vi "Entry.vi"(8 "error in (no error)":errorcluster, 11 "New State":refnum<class "Command State Actor.lvclass">) -> (0 "error out":errorcluster, 3 "State out":refnum<class "Command State Actor.lvclass">)   [LabVIEW 2013, in "Command State Actor.lvlib" / "Command State Actor.lvclass"]
doc: "This is an abstract method. Override this method to define the behavior when you enter the state."
uses:
  Command State Actor.lvclass
  <vilib>/ni/Actors/State Actor/State Actor/State Actor.lvclass
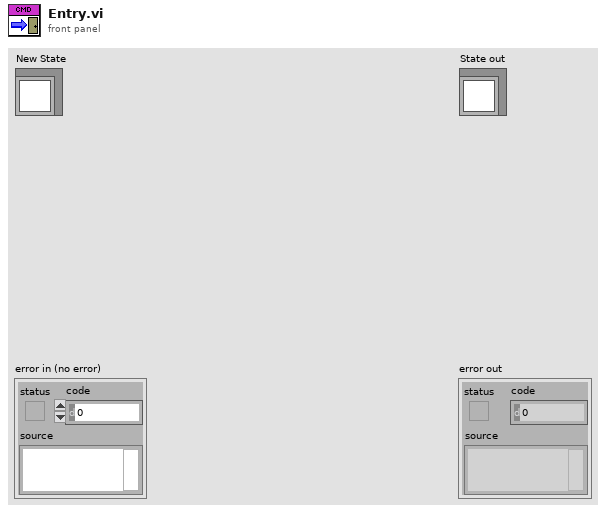
[diagram p1: front panel]
types:
  T1 = typedef "Command State Actor.lvlib/Command State Actor.lvclass/Command Status.ctl" = cluster{"CurrentCommandState":T2, "Command Name":string, "Current State Status":T3, "Command Start Time":timestamp, "Command End Time":timestamp, "Previous State Status":T3}
  T2 = typedef "Command State Actor.lvlib/Command State Actor.lvclass/Command States.ctl" = enum16{"NotStarted", "Starting", "Started", "Executing", "Completing", "Completed", "Stopping", "Stopped"}
  T3 = typedef "Command Actor.lvlib/Command States.lvclass/State Status.ctl" = cluster{"State Name":string, "State Entry Time":timestamp, "State Exit Time":timestamp}
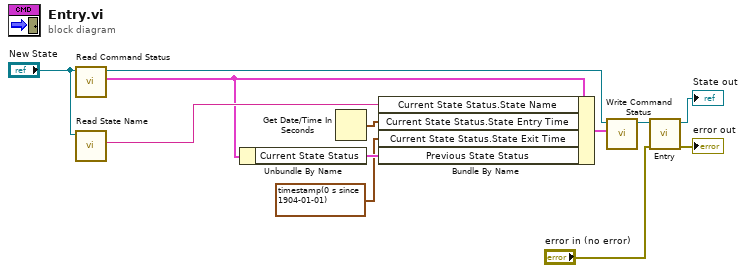
[diagram p0: block diagram]
diagram:
  n1 = call-dynamic "Read Command Status.vi"("Command in"="New State") -> ("Command Status"=w3:T1, "Command out"=w9:refnum<class "Command State Actor.lvclass">)  [unwired: 8 in, 1 out]
  n2 = call-dynamic "Read State Name.vi"("Command State Actor in"="New State") -> ("State Name"=w6:string)  [unwired: 8 in, 2 out]
  n3 = Unbundle By Name(w3) -> ("Current State Status"=w2:T3)
  n4 = Get Date/Time In Seconds() -> (seconds since 1Jan1904=w5:timestamp)
  n5 = Bundle By Name(cluster=w3, "Current State Status.State Name"=w6, "Current State Status.State Entry Time"=w5, "Current State Status.State Exit Time"=timestamp(0 s since 1904-01-01), "Previous State Status"=w2) -> (w7:T1)
  n6 = call-dynamic "Write Command Status.vi"("Command Status"=w7, "Command in"=w9) -> ("Command out"=w8:refnum<class "Command State Actor.lvclass">)  [unwired: 8 in, 1 out]
  n7 = call-parent "Entry.vi"("error in (no error)"="error in (no error)", "New State"=w8) -> ("error out"=→"error out":errorcluster, "State out"=→"State out":refnum<class "Command State Actor.lvclass">)  [unwired: 8 in]
